vi "arduinoTempsBad.vi"() -> ()   [LabVIEW 2023]
uses:
  <vilib>/Instr/_visa.llb/VISA Configure Serial Port (Instr).vi
panel:
  in  "stop":bool=TRUE
  out "temp4":dbl
  out "temp3":dbl
  out "temp2":dbl
  out "temp1":dbl
  out "error out":errorcluster
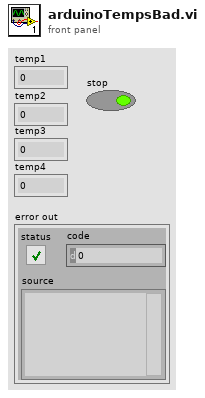
[diagram p1: front panel]
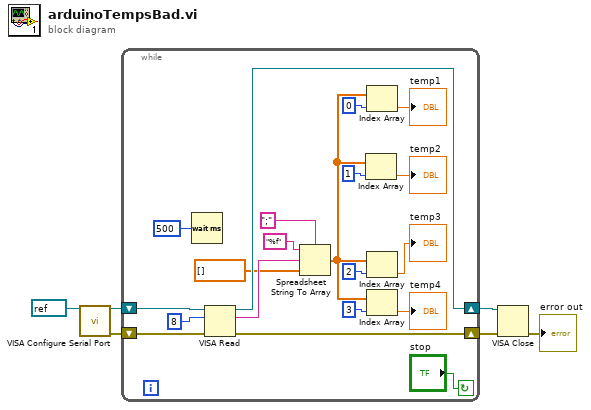
[diagram p0: block diagram]
diagram:
  n1 = call-poly "VISA Configure Serial Port"("VISA resource name"=refnum<visa-resource-name> refnum) -> ("VISA resource name out"=w4:refnum<visa-resource-name>, "error out"=w5:errorcluster)  [unwired: 13 in]
  n2 = while {
    shift-right: [w23] -> w2
    shift-left: w5 -> [w26]
    shift-right: [w24] -> w3
    shift-left: w4 -> [w25]
    stop <- "stop" continue-if-true
    n3 = Wait (ms)(milliseconds to wait=u32 500) -> ()  [unwired: 1 out]
    n4 = VISA Read(VISA resource name=w25, byte count=u32 8, error in (no error)=w26) -> (VISA resource name out=w24:refnum<visa-resource-name>, read buffer=w22:string, error out=w23:errorcluster)  [unwired: 1 out]
    n5 = Spreadsheet String To Array(delimiter (Tab)=";", format string="%f", spreadsheet string=w22, array type (2D Dbl)=dbl[] []) -> (array=w19:dbl[])
    n6 = Index Array(array=w19, index=1) -> (element=→"temp2":dbl)
    n7 = Index Array(array=w19, index=0) -> (element=→"temp1":dbl)
    n8 = Index Array(array=w19, index=2) -> (element=→"temp3":dbl)
    n9 = Index Array(array=w19, index=3) -> (element=→"temp4":dbl)
  }
  n10 = VISA Close(VISA resource name=w3, error in (no error)=w2) -> (error out=→"error out":errorcluster)
